vi "BoxNetworking.vi"   [LabVIEW 2023]
uses:
  BoxNetworkingGlobal.vi
  <vilib>/Rock Robotics/Network Tables/NT Write Boolean.vi
  <vilib>/Rock Robotics/Network Tables/NT Write String.vi
  <vilib>/Rock Robotics/Network Tables/NT Write Number.vi
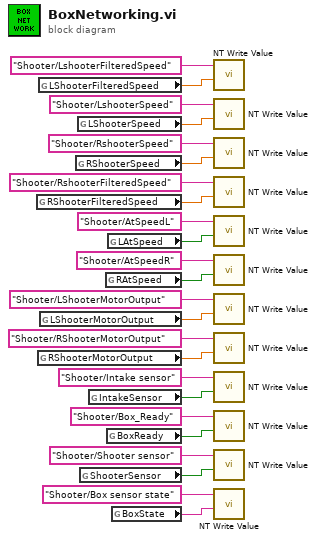
[diagram p0: block diagram]
diagram:
  n1 = global read "BoxNetworkingGlobal.vi" "RShooterFilteredSpeed"() -> (w9:dbl)
  n2 = global read "BoxNetworkingGlobal.vi" "RShooterMotorOutput"() -> (w1:dbl)
  n3 = global read "BoxNetworkingGlobal.vi" "LShooterFilteredSpeed"() -> (w15:dbl)
  n4 = global read "BoxNetworkingGlobal.vi" "LShooterMotorOutput"() -> (w3:dbl)
  n5 = global read "BoxNetworkingGlobal.vi" "RShooterSpeed"() -> (w11:dbl)
  n6 = global read "BoxNetworkingGlobal.vi" "LShooterSpeed"() -> (w13:dbl)
  n7 = global read "BoxNetworkingGlobal.vi" "ShooterSensor"() -> (w21:bool)
  n8 = global read "BoxNetworkingGlobal.vi" "IntakeSensor"() -> (w17:bool)
  n9 = global read "BoxNetworkingGlobal.vi" "RAtSpeed"() -> (w5:bool)
  n10 = global read "BoxNetworkingGlobal.vi" "BoxReady"() -> (w19:bool)
  n11 = global read "BoxNetworkingGlobal.vi" "LAtSpeed"() -> (w7:bool)
  n12 = global read "BoxNetworkingGlobal.vi" "BoxState"() -> (w24:string)
  n13 = call-poly <vilib>:"NT Write Value.vi"("value"=w15, "name"="Shooter/LshooterFilteredSpeed") -> ()  [unwired: 9 in, 1 out]
  n14 = call-poly <vilib>:"NT Write Value.vi"("value"=w13, "name"="Shooter/LshooterSpeed") -> ()  [unwired: 9 in, 1 out]
  n15 = call-poly <vilib>:"NT Write Value.vi"("value"=w11, "name"="Shooter/RshooterSpeed") -> ()  [unwired: 9 in, 1 out]
  n16 = call-poly <vilib>:"NT Write Value.vi"("value"=w9, "name"="Shooter/RshooterFilteredSpeed") -> ()  [unwired: 9 in, 1 out]
  n17 = call-poly <vilib>:"NT Write Value.vi"("value"=w7, "name"="Shooter/AtSpeedL") -> ()  [unwired: 9 in, 1 out]
  n18 = call-poly <vilib>:"NT Write Value.vi"("value"=w5, "name"="Shooter/AtSpeedR") -> ()  [unwired: 9 in, 1 out]
  n19 = call-poly <vilib>:"NT Write Value.vi"("value"=w3, "name"="Shooter/LShooterMotorOutput") -> ()  [unwired: 9 in, 1 out]
  n20 = call-poly <vilib>:"NT Write Value.vi"("value"=w1, "name"="Shooter/RShooterMotorOutput") -> ()  [unwired: 9 in, 1 out]
  n21 = call-poly <vilib>:"NT Write Value.vi"("value"=w17, "name"="Shooter/Intake sensor") -> ()  [unwired: 9 in, 1 out]
  n22 = call-poly <vilib>:"NT Write Value.vi"("value"=w19, "name"="Shooter/Box_Ready") -> ()  [unwired: 9 in, 1 out]
  n23 = call-poly <vilib>:"NT Write Value.vi"("value"=w21, "name"="Shooter/Shooter sensor") -> ()  [unwired: 9 in, 1 out]
  n24 = call-poly <vilib>:"NT Write Value.vi"("value"=w24, "name"="Shooter/Box sensor state") -> ()  [unwired: 9 in, 1 out]
